vi "ST5520_CMD.vi"() -> ()   [LabVIEW 2020]
uses:
  <vilib>/Instr/_visa.llb/VISA Find Search Mode.ctl
  VG/R_VG.vi
  <vilib>/Utility/inputDevices.llb/keyboardAcquire.vi
panel:
  out "errout":errorcluster caption="sortie d'erreur"
  out "keys pressed":T1(array[ring]) caption="touches enfoncées"
  out "Resistance Ohms":dbl
  in  "Arrêter":bool
  in  "errin":errorcluster caption="entrée d'erreur (pas d'erreur)"
  out "VISA OUT":refnum<visa-resource-name>
  out "DATA OUT":string
  # "DATA OUT"
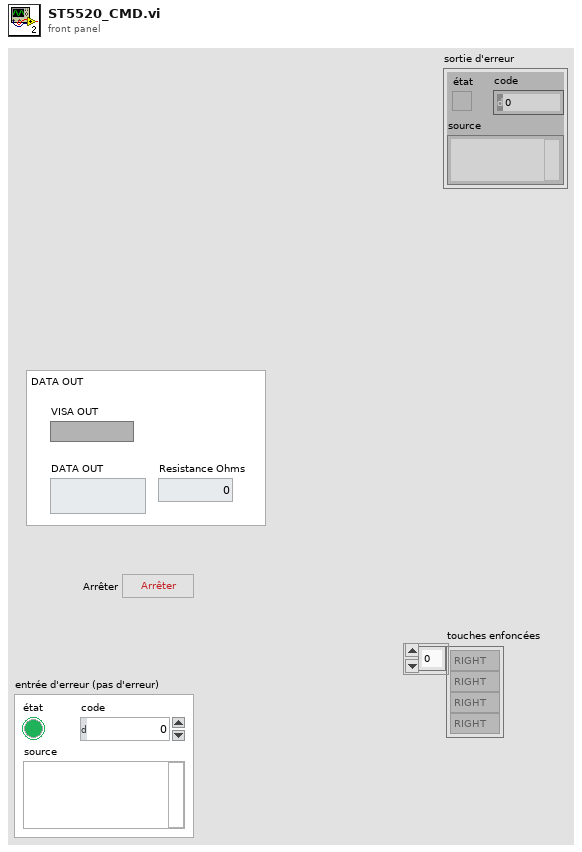
[diagram p1: front panel]
types:
  T1 = enum16{"0", "1", "2", "3", "4", "5", "6", "7", "8", "9", "A", "B", "C", "D", "E", "F", "G", "H", "I", "J", "K", "L", "M", "N", "O", "P", "Q", "R", "S", "T", "U", "V", "W", "X", "Y", "Z", "F1", "F2", "F3", "F4", "F5", "F6", "F7", "F8", "F9", "F10", "F11", "F12", "F13", "F14", "F15", "ADD", "BACK", "BACKSLASH", "CAPITAL", "COMMA", "DECIMAL", "DELETE", "DIVIDE", "DOWN", "END", "EQUALS", "ESCAPE", "GRAVE (`)", "HOME", "INSERT", "LBRACKET", "LCONTROL", "LEFT", "L ALT", "LSHIFT", "LWIN", "MINUS", "MULTIPLY", "NEXT", "NUMLOCK", "NUMPAD_0", "NUMPAD_1", "NUMPAD_2", "NUMPAD_3", "NUMPAD_4", "NUMPAD_5", "NUMPAD_6", "NUMPAD_7", "NUMPAD_8", "NUMPAD_9", "PAUSE", "PERIOD", "PRIOR (PG UP)", "RBRACKET", "RCONTROL", "RETURN", "RIGHT", "R ALT", "RSHIFT", "RWIN", "SCROLL", "SEMICOLON", "SLASH", "SPACE", "SUBTRACT", "TAB", "UP", "ENTER (num pad)", "' (quote)"}[]
  T2 = typedef "VISA Find Search Mode.ctl" = u32
  T3 = enum16{"0", "1", "2", "3", "4", "5", "6", "7", "8", "9", "A", "B", "C", "D", "E", "F", "G", "H", "I", "J", "K", "L", "M", "N", "O", "P", "Q", "R", "S", "T", "U", "V", "W", "X", "Y", "Z", "F1", "F2", "F3", "F4", "F5", "F6", "F7", "F8", "F9", "F10", "F11", "F12", "F13", "F14", "F15", "ADD", "BACK", "BACKSLASH", "CAPITAL", "COMMA", "DECIMAL", "DELETE", "DIVIDE", "DOWN", "END", "EQUALS", "ESCAPE", "GRAVE (`)", "HOME", "INSERT", "LBRACKET", "LCONTROL", "LEFT", "L ALT", "LSHIFT", "LWIN", "MINUS", "MULTIPLY", "NEXT", "NUMLOCK", "NUMPAD_0", "NUMPAD_1", "NUMPAD_2", "NUMPAD_3", "NUMPAD_4", "NUMPAD_5", "NUMPAD_6", "NUMPAD_7", "NUMPAD_8", "NUMPAD_9", "PAUSE", "PERIOD", "PRIOR (PG UP)", "RBRACKET", "RCONTROL", "RETURN", "RIGHT", "R ALT", "RSHIFT", "RWIN", "SCROLL", "SEMICOLON", "SLASH", "SPACE", "SUBTRACT", "TAB", "UP", "ENTER (num pad)", "' (quote)"}
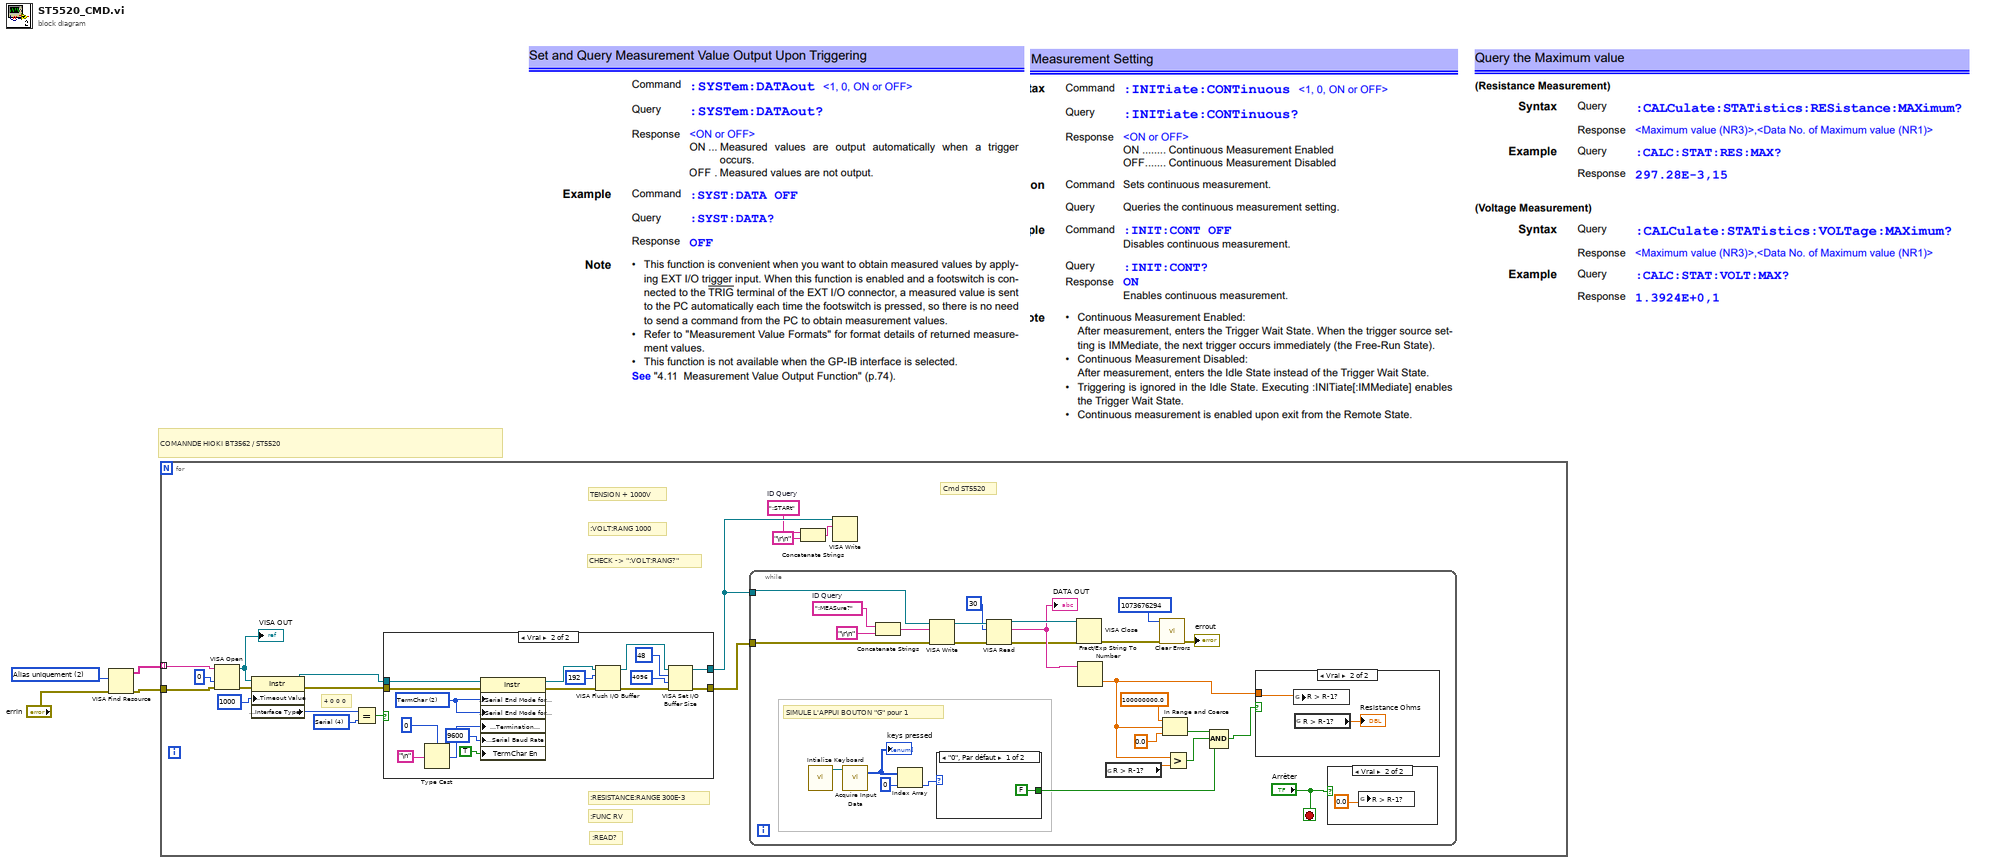
[diagram p0: block diagram]
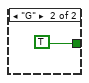
[diagram p2: hidden frame]
diagram:
  w4 = T2 2 items=["Noms canoniques uniquement"=0, "Alias uniquement"=2, "Inclure les alias correspondants"=3, "Inclure tous les alias"=4] ("Search Mode")
  # "COMANNDE HIOKI BT3562 / ST5520"
  n1 = VISA Find Resource(8:"errin", 10:w4) -> (0:w2:errorcluster, 3:w3:string[])  [unwired: 1 in, 1 out]
  n2 = for {
    tunnel: w3 -> [w14] mode=indexing
    tunnel: w2 -> [w13]
    w6 = ":STARt"  # ID Query
    w16 = u16 4 items=["GPIB"=1, "VXI"=2, "GPIB-VXI"=3, "Serial"=4, "PXI"=5, "TCPIP"=6, "USB"=7] ("Interface Information:Interface Type")
    # ":READ?"
    # ":FUNC RV"
    # ":RESISTANCE:RANGE 300E-3"
    # "Cmd ST5520"
    # "CHECK -> \":VOLT:RANG?\""
    # ":VOLT:RANG 1000"
    # "TENSION + 1000V"
    # "4 0 0 0"
    n3 = VISA Open(access mode=u32 0, error in (no error)=w13, VISA resource name=w14) -> (VISA resource name=w18:refnum<visa-resource-name>, error out=w17:errorcluster)  [unwired: 2 in]
    "VISA OUT" <- w18
    n4 = property class="Instr"(reference=w18, error in=w17, "General Settings:Timeout Value"=u32 1000) -> (reference out=w11:refnum<visa-resource-name>, error out=w10:errorcluster, "Interface Information:Interface Type"=w15:u16)
    n5 = Equal?(x=w15, y=w16) -> (x = y?=w12:bool)
    n6 = case shown="Vrai" w12 {
      tunnel: [w53 w68] -> w8
      tunnel: [w54 w65] -> w9
      tunnel: w11 -> [w53 w70]
      tunnel: w10 -> [w54 w71]
      frame False {
        # "EDIT: Remove interfaces not supported by your instrument."
        # "GPIB, TCP/IP, and USB Interface"
      }
      frame True {
        w58 = u16 2 items=["None", "LastBit", "TermChar"] ("Serial Settings:Serial End Mode for Reads")
        n7 = Type Cast(type=u8 0, x="\n" ("Line Feed Constant")) -> (*(type *) &x=w57:u8)
        n8 = property class="Instr"(reference=w70, error in=w71, "Serial Settings:Serial End Mode for Reads"=w58, "Serial Settings:Serial End Mode for Writes"=w58, "Message Based Settings:Termination Character"=w57, "Serial Settings:Serial Baud Rate"=u32 9600 ("Serial Settings:Baud Rate"), "TermChar En"=TRUE ("Message Based Settings:Termination Character Enable")) -> (reference out=w64:refnum<visa-resource-name>, error out=w67:errorcluster)
        n9 = VISA Flush I/O Buffer(VISA resource name=w64, mask (16)=u16 192, error in (no error)=w67) -> (VISA resource name out=w69:refnum<visa-resource-name>, error out=w66:errorcluster)
        n10 = VISA Set I/O Buffer Size(VISA resource name=w69, mask (16)=u16 48, size (4096)=u32 4096 ("size (0)"), error in (no error)=w66) -> (VISA resource name out=w68:refnum<visa-resource-name>, error out=w65:errorcluster)
      }
    }
    n11 = while {
      tunnel: w9 -> [w36]
      tunnel: w8 -> [w37]
      stop <- "Arrêter" stop-if-true
      w47 = ":MEASure?"  # ID Query
      # "SIMULE L'APPUI BOUTON \"G\" pour 1"
      n12 = call <vilib>:"Intialize Keyboard.vi"() -> ("device ID"=w34:refnum<k1>)  [unwired: 10 in, 1 out]
      n13 = call-poly <vilib>:"Acquire Input Data.vi"("device ID"=w34) -> ("keys pressed"=w25:T1)  [unwired: 16 in, 2 out]
      "keys pressed" <- w25
      n14 = Concatenate Strings(w47, "\r\n") -> (w41:string)
      n15 = Index Array(array=w25, index=0 ("indice")) -> (element=w23:T3)
      n16 = VISA Write(VISA resource name=w37, write buffer=w41, error in (no error)=w36) -> (VISA resource name out=w46:refnum<visa-resource-name>, error out=w45:errorcluster)  [unwired: 1 out]
      n17 = case shown="\"0\", Par défaut" w23 {
        tunnel: [FALSE TRUE] -> w26
        frame "0", Default {
        }
        frame "G" {
        }
      }
      n18 = VISA Read(VISA resource name=w46, byte count=u32 30 ("nombre d'octets"), error in (no error)=w45) -> (VISA resource name out=w43:refnum<visa-resource-name>, read buffer=w40:string, error out=w35:errorcluster)  [unwired: 1 out]
      "DATA OUT" <- w40
      n19 = VISA Close(VISA resource name=w43, error in (no error)=w35) -> (error out=w44:errorcluster)
      n20 = Fract/Exp String To Number(string=w40) -> (number=w31:dbl)  [unwired: 3 in, 1 out]
      n21 = global read "R_VG.vi" "R > R-1?"() -> (w30:dbl)
      n22 = call <vilib>:"Clear Errors.vi"("error in (no error)"=w44, "specific error code to clear (0: all)"=1073676294) -> ("error out"=→"errout":errorcluster)  [unwired: 4 in, 1 out]
      n23 = In Range and Coerce(upper limit=100000000.0 ("limite supérieure"), x=w31, lower limit=0.0 ("limite inférieure")) -> (In Range?=w29:bool)  [unwired: 1 out]
      n24 = Greater?(x=w31, y=w30) -> (0:w28:bool)
      n25 = Compound Arithmetic op=AND ("Opérateur arithmétique")(w29, w28, w26) -> (w27:bool)
      n26 = case shown="Vrai" w27 {
        tunnel: w31 -> [_ w52]
        frame False {
        }
        frame True {
          n27 = global write "R_VG.vi" "R > R-1?"(w52) -> ()
          n28 = global read "R_VG.vi" "R > R-1?"() -> (→"Resistance Ohms":dbl)
        }
      }
      n29 = case shown="Vrai" "Arrêter" {
        frame False {
        }
        frame True {
          n30 = global write "R_VG.vi" "R > R-1?"(0.0 ("R > R-1?")) -> ()
        }
      }
    }
    n31 = Concatenate Strings(w6, "\r\n") -> (w7:string)
    n32 = VISA Write(VISA resource name=w8, write buffer=w7) -> ()  [unwired: 1 in, 3 out]
  }
